vi "Begin.vi"() -> (0 "error out":errorcluster)   [LabVIEW 2013]
doc: "Called before other user functions, this VI is expected to open initial I/O refnums, load in file data, and do all program initialization. Notice that the <B>error out</B> terminal is simply used for data flow. Wiring it to other structures or subVIs ensures that this VI runs first."
uses:
  <vilib>/Rock Robotics/WPI/DriverStation/WPI_DriverStationRobotMode2.ctl
  <vilib>/Rock Robotics/WPI/Joystick/WPI_JoystickDeviceEnum.ctl
  <vilib>/Rock Robotics/SystemInterfaces/DIO/FPGA_DIOPWMChannel.ctl
  <vilib>/Rock Robotics/SystemInterfaces/DIO/FPGA_DIOChannel.ctl
  <vilib>/Rock Robotics/WPI/Encoder/WPI_EncoderType.ctl
  <vilib>/Rock Robotics/WPI/Solenoid/WPI_SolenoidChannel.ctl
  <vilib>/Rock Robotics/SystemInterfaces/AI/FPGA_AIGyroChannel.ctl
  <vilib>/Rock Robotics/SystemInterfaces/DIO/FPGA_DIORelayChannel.ctl
  Robot Global Data.vi
  <vilib>/Rock Robotics/WPI/Counter/WPI_CounterDigitalInputToDigitalSource.vi
  <vilib>/Rock Robotics/WPI/MotorControl/WPI_MotorControlOpen Talon.vi
  <vilib>/Rock Robotics/WPI/Solenoid/WPI_SolenoidOpenSingle.vi
  <vilib>/Rock Robotics/WPI/Compressor/WPI_CompressorGetSetRefNum.vi
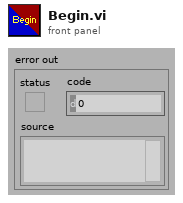
[diagram p1: front panel]
types:
  T1 = typedef "FPGA_DIORelayChannel.ctl" = enum8{"Relay 1", "Relay 2", "Relay 3", "Relay 4", "Relay 5", "Relay 6", "Relay 7", "Relay 8", "Invalid"}
  T2 = typedef "FPGA_DIOChannel.ctl" = enum8{"DIO 1", "DIO 2", "DIO 3", "DIO 4", "DIO 5", "DIO 6", "DIO 7", "DIO 8", "DIO 9", "DIO 10", "DIO 11", "DIO 12", "DIO 13", "DIO 14", "Invalid"}
  T3 = typedef "WPI_SolenoidChannel.ctl" = enum8{"Solenoid 1", "Solenoid 2", "Solenoid 3", "Solenoid 4", "Solenoid 5", "Solenoid 6", "Solenoid 7", "Solenoid 8", "Invalid"}
  T4 = typedef "FPGA_DIOPWMChannel.ctl" = enum8{"PWM 1", "PWM 2", "PWM 3", "PWM 4", "PWM 5", "PWM 6", "PWM 7", "PWM 8", "PWM 9", "PWM 10", "Invalid"}
  T5 = typedef "FPGA_AIGyroChannel.ctl" = enum8{"AI 1", "AI 2", "Invalid"}
  T6 = typedef "WPI_EncoderType.ctl" = enum16{"1x", "2x", "4x"}
  T7 = typedef "WPI_JoystickDeviceEnum.ctl" = enum16{"USB 1", "USB 2", "USB 3", "USB 4", "Kinect 1", "Kinect 2"}
  T8 = typedef "WPI_DriverStationRobotMode2.ctl" = enum16{"Autonomous Disabled", "Autonomous Enabled", "Teleop Disabled", "Teleop Enabled", "Timeout", "Finish", "Test Disabled", "Test Enabled"}
  T9 = typedef "WPI_JoystickDevRef.ctl" = cluster{"Device":T7}
  T10 = typedef "WPI_DigitalInputDevRef.ctl" = cluster{"DevStatus":errorcluster, "DIO Channel":T2, "Digital Module":T11}
  T11 = typedef "FPGA_TypedefDigitalModule.ctl" = enum16{"Digital Module 1", "Digital Module 2"}
  T12 = typedef "FPGA_CounterEncoderSourceConvertionLVSourceType.ctl" = cluster{"DevStatus":errorcluster, "AnalogTriggerMode?":bool, "DigitalMode":cluster{"Digital Module":T11, "DIO Channel":T13}, "AnalogTriggerMode":cluster{"AnalogTriggerIndex":T14, "OutputType":T15}}
  T13 = typedef "FPGA_DIODigitalSourceChannel.ctl" = enum8{"DIO 1", "DIO 2", "DIO 3", "DIO 4", "DIO 5", "DIO 6", "DIO 7", "DIO 8", "DIO 9", "DIO 10", "DIO 11", "DIO 12", "DIO 13", "DIO 14", "Disabled"}
  T14 = typedef "FPGA_AnalogTriggerIndex.ctl" = enum8{"Trig 0", "Trig 1", "Trig 2", "Trig 3", "Trig 4", "Trig 5", "Trig 6", "Trig 7", "Invalid"}
  T15 = typedef "FPGA_AnalogTriggerOutType.ctl" = enum16{"InWindow", "TriggerState", "Rising", "Falling"}
  T16 = typedef "WPI_EncoderDevRef.ctl" = cluster{"DevStatus":errorcluster, "EncoderIndex":T17, "CounterIndex":T18, "DistancePerCount":dbl, "Decoding Type":T6}
  T17 = typedef "FPGA_EncoderIdx.ctl" = enum8{"Enc 0", "Enc 1", "Enc 2", "Enc 3", "Invalid"}
  T18 = typedef "FPGA_CounterCtrSystemIndex.ctl" = enum8{"Ctr 0", "Ctr 1", "Ctr 2", "Ctr 3", "Ctr 4", "Ctr 5", "Ctr 6", "Ctr 7", "Invalid"}
  T19 = typedef "WPI_MotorControlDeviceRef.ctl" = cluster{"DeviceStatus":errorcluster, "Type":enum16{"PWM", "CAN"}, "PWM":cluster{"Digital Module":T11, "PWM Channel":T4, "DeadBand":T20}, "CAN":cluster{"Device Number":u8, "Control Mode":T21, "Semaphore":T22, "Max Vout":dbl}, "Invert":bool, "TransformRef":T23, "InvTransformRef":T23}
  T20 = typedef "WPI_PWMDeadband.ctl" = cluster{"Name":string, "maxPositivePwm":i32, "minPositivePwm":i32, "centerPwm":i32, "maxNegativePwm":i32, "minNegativePwm":i32, "angularRange":u16}
  T21 = typedef "WPI_CANJaguar_ControlMode.ctl" = enum8{"Percent VBus", "Current", "Speed", "Position", "Voltage"}
  T22 = typedef "Semaphore RefNum" = refnum<k1>
  T23 = typedef "WPI_PWMTransform_ConPane.ctl" = refnum<vi>
  T24 = typedef "WPI_GyroDevRef.ctl" = cluster{"DevStatus":errorcluster, "Analog Module":T25, "Analog Channel":T26, "Offset":dbl, "Gain (VoltsPerDegree/Second)":dbl}
  T25 = typedef "FPGA_TypedefAnalogModule.ctl" = enum16{"Analog Module 1", "Analog Module 2"}
  T26 = typedef "FPGA_AIChannel.ctl" = enum8{"AI 1", "AI 2", "AI 3", "AI 4", "AI 5", "AI 6", "AI 7", "AI 8", "Invalid"}
  T27 = typedef "WPI_SolenoidDevRef.ctl" = cluster{"DevStatus":errorcluster, "Solenoid Module":T28, "Forward Solenoid Channel":T3, "Reverse Solenoid Channel":T3}
  T28 = typedef "FPGA_TypedefSolenoidModule.ctl" = enum16{"Solenoid Module 1", "Solenoid Module 2"}
  T29 = typedef "WPI_CompressorDevRef.ctl" = cluster{"DevStatus":errorcluster, "DigitalInputDevRef":T10, "RelayDevRef":T30}
  T30 = typedef "WPI_RelayDevRef.ctl" = cluster{"DevStatus":errorcluster, "Relay Channel":T1, "Digital Module":T11, "Relay Direction":T31}
  T31 = typedef "WPI_RelayDirection.ctl" = enum16{"Both directions", "Forward only", "Reverse only"}
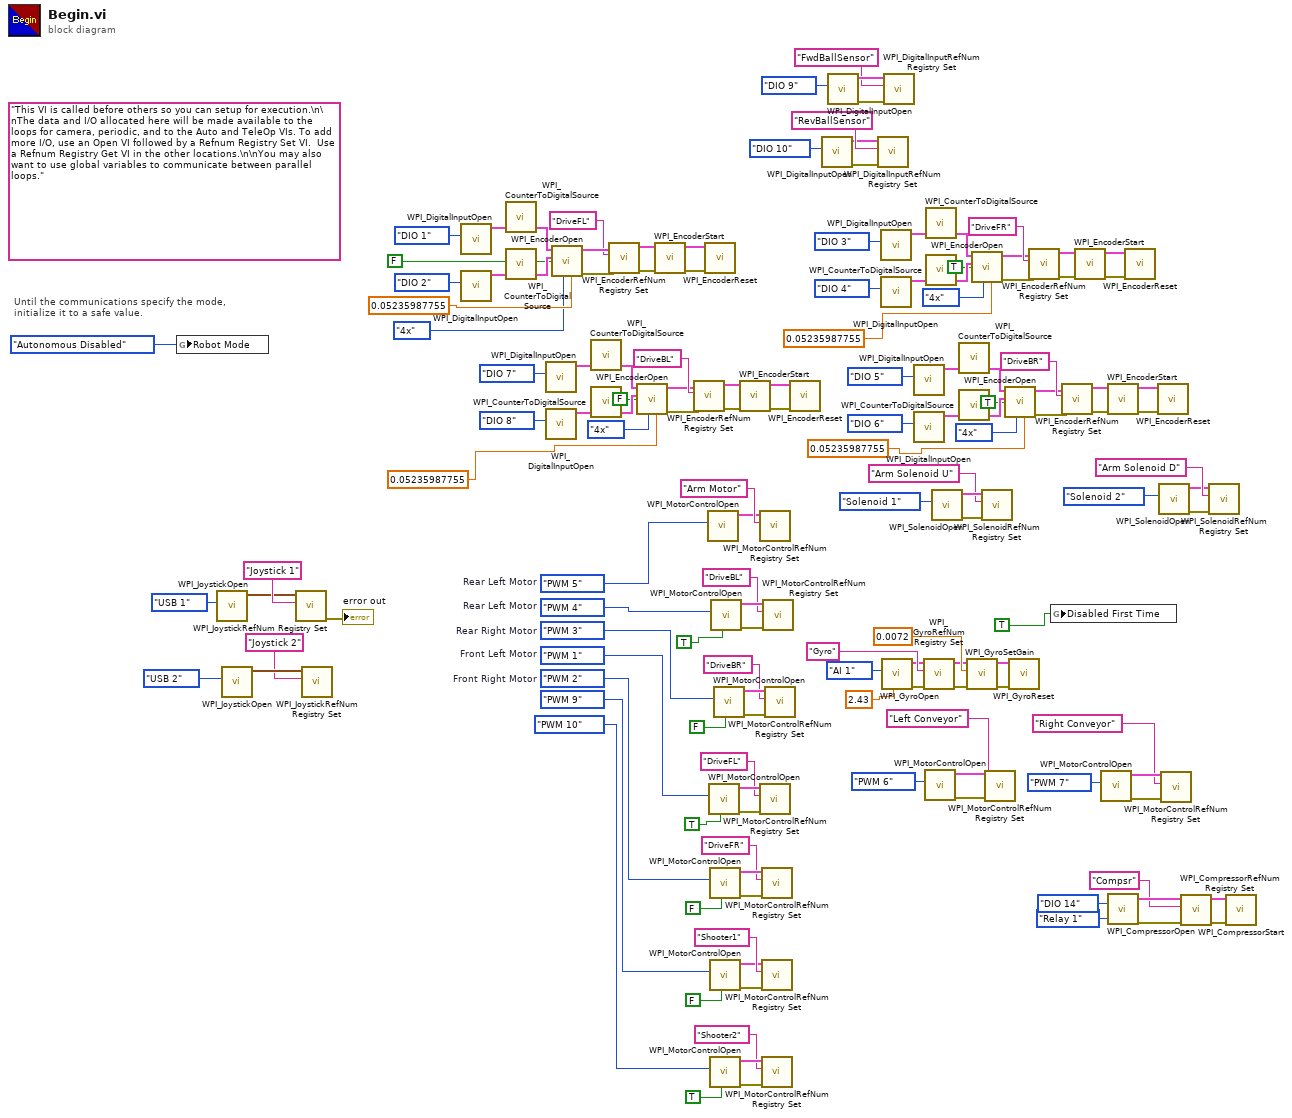
[diagram p0: block diagram]
diagram:
  w58 = FPGA_DIOPWMChannel."PWM 5"  # Rear Left Motor
  w67 = FPGA_DIOPWMChannel."PWM 2"  # Front Right Motor
  w68 = FPGA_DIOPWMChannel."PWM 1"  # Front Left Motor
  w69 = FPGA_DIOPWMChannel."PWM 3"  # Rear Right Motor
  w70 = FPGA_DIOPWMChannel."PWM 4"  # Rear Left Motor
  (unwired) "This VI is called before others so you can setup for execution.\n\nThe data and I/O allocated here will be made available to the loops for camera, periodic, and to the Auto and TeleOp VIs. To add more I/O, use an Open VI followed by a Refnum Registry Set VI.  Use a Refnum Registry Get VI in the other locations.\n\nYou may also want to use global variables to communicate between parallel loops."
  # "Until the communications specify the mode,\ninitialize it to a safe value."
  n1 = global write "Robot Global Data.vi" "Robot Mode"(WPI_DriverStationRobotMode2."Autonomous Disabled" ("Robot Mode")) -> ()
  n2 = call <vilib>:"WPI_JoystickOpen.vi"("JoystickDevice"=WPI_JoystickDeviceEnum."USB 1") -> ("JoystickDevRef"=w145:T9)  [unwired: 10 in]
  n3 = call <vilib>:"WPI_JoystickOpen.vi"("JoystickDevice"=WPI_JoystickDeviceEnum."USB 2") -> ("JoystickDevRef"=w141:T9)  [unwired: 10 in]
  n4 = call <vilib>:"WPI_JoystickRefNum Registry Set.vi"("refnum name"="Joystick 1", "JoystickDevRef"=w145) -> ("error out"=→"error out":errorcluster)  [unwired: 8 in, 1 out]
  n5 = call <vilib>:"WPI_JoystickRefNum Registry Set.vi"("refnum name"="Joystick 2", "JoystickDevRef"=w141) -> ()  [unwired: 8 in, 2 out]
  n6 = call <vilib>:"WPI_DigitalInputOpen.vi"("DIO Channel"=FPGA_DIOChannel."DIO 1") -> ("DigitalInputDevRef"=w113:T10)  [unwired: 9 in, 1 out]
  n7 = call <vilib>:"WPI_DigitalInputOpen.vi"("DIO Channel"=FPGA_DIOChannel."DIO 2") -> ("DigitalInputDevRef"=w116:T10)  [unwired: 9 in, 1 out]
  n8 = call-poly <vilib>:"WPI_CounterToDigitalSource.vi"("DigitalInputDevRef"=w113) -> ("Digital Source"=w114:T12)  [unwired: 6 in]
  n9 = call-poly <vilib>:"WPI_CounterToDigitalSource.vi"("DigitalInputDevRef"=w116) -> ("Digital Source"=w115:T12)  [unwired: 6 in]
  n10 = call <vilib>:"WPI_DigitalInputOpen.vi"("DIO Channel"=FPGA_DIOChannel."DIO 7") -> ("DigitalInputDevRef"=w137:T10)  [unwired: 9 in, 1 out]
  n11 = call <vilib>:"WPI_DigitalInputOpen.vi"("DIO Channel"=FPGA_DIOChannel."DIO 8") -> ("DigitalInputDevRef"=w134:T10)  [unwired: 9 in, 1 out]
  n12 = call <vilib>:"WPI_EncoderOpen.vi"("DistancePerCount"=0.05235987755, "Decoding Type"=WPI_EncoderType."4x", "Invert Direction (False)"=FALSE, "BSource"=w115, "ASource"=w114) -> ("error out"=w123:errorcluster, "EncoderDevRef"=w122:T16)  [unwired: 5 in]
  n13 = call-poly <vilib>:"WPI_CounterToDigitalSource.vi"("DigitalInputDevRef"=w137) -> ("Digital Source"=w136:T12)  [unwired: 6 in]
  n14 = call-poly <vilib>:"WPI_CounterToDigitalSource.vi"("DigitalInputDevRef"=w134) -> ("Digital Source"=w135:T12)  [unwired: 6 in]
  n15 = call <vilib>:"WPI_EncoderRefNum Registry Set.vi"("error in (no error)"=w123, "refnum name"="DriveFL", "EncoderDevRef"=w122) -> ("error out"=w125:errorcluster, "EncoderDevRef"=w124:T16)  [unwired: 7 in]
  n16 = call <vilib>:"WPI_EncoderOpen.vi"("DistancePerCount"=0.05235987755, "Decoding Type"=WPI_EncoderType."4x", "Invert Direction (False)"=FALSE, "BSource"=w135, "ASource"=w136) -> ("error out"=w128:errorcluster, "EncoderDevRef"=w129:T16)  [unwired: 5 in]
  n17 = call <vilib>:"WPI_EncoderStart.vi"("error in (no error)"=w125, "EncoderDevRef"=w124) -> ("error out"=w121:errorcluster, "EncoderDevRef"=w120:T16)  [unwired: 8 in]
  n18 = call <vilib>:"WPI_EncoderRefNum Registry Set.vi"("error in (no error)"=w128, "refnum name"="DriveBL", "EncoderDevRef"=w129) -> ("error out"=w126:errorcluster, "EncoderDevRef"=w127:T16)  [unwired: 7 in]
  n19 = call <vilib>:"WPI_EncoderReset.vi"("error in (no error)"=w121, "EncoderDevRef"=w120) -> ()  [unwired: 8 in, 2 out]
  n20 = call-poly <vilib>:"WPI_MotorControlOpen.vi"("PWM Channel"=w58) -> ("MotorControlDeviceRef"=w56:T19)  [unwired: 9 in, 1 out]
  n21 = call-poly <vilib>:"WPI_MotorControlOpen.vi"("Invert"=TRUE, "PWM Channel"=w68) -> ("error out"=w77:errorcluster, "MotorControlDeviceRef"=w78:T19)  [unwired: 8 in]
  n22 = call-poly <vilib>:"WPI_MotorControlOpen.vi"("Invert"=FALSE, "PWM Channel"=w67) -> ("error out"=w75:errorcluster, "MotorControlDeviceRef"=w76:T19)  [unwired: 8 in]
  n23 = call-poly <vilib>:"WPI_MotorControlOpen.vi"("Invert"=FALSE, "PWM Channel"=FPGA_DIOPWMChannel."PWM 9") -> ("error out"=w31:errorcluster, "MotorControlDeviceRef"=w30:T19)  [unwired: 8 in]
  n24 = call-poly <vilib>:"WPI_MotorControlOpen.vi"("Invert"=TRUE, "PWM Channel"=FPGA_DIOPWMChannel."PWM 10") -> ("error out"=w28:errorcluster, "MotorControlDeviceRef"=w29:T19)  [unwired: 8 in]
  n25 = call-poly <vilib>:"WPI_MotorControlOpen.vi"("Invert"=TRUE, "PWM Channel"=w70) -> ("error out"=w81:errorcluster, "MotorControlDeviceRef"=w82:T19)  [unwired: 8 in]
  n26 = call-poly <vilib>:"WPI_MotorControlOpen.vi"("Invert"=FALSE, "PWM Channel"=w69) -> ("error out"=w79:errorcluster, "MotorControlDeviceRef"=w80:T19)  [unwired: 8 in]
  n27 = call <vilib>:"WPI_EncoderStart.vi"("error in (no error)"=w126, "EncoderDevRef"=w127) -> ("error out"=w130:errorcluster, "EncoderDevRef"=w131:T16)  [unwired: 8 in]
  n28 = call <vilib>:"WPI_MotorControlRefNum Registry Set.vi"("refnum name"="Arm Motor", "MotorControlDevRef"=w56) -> ()  [unwired: 8 in, 2 out]
  n29 = call <vilib>:"WPI_MotorControlRefNum Registry Set.vi"("error in (no error)"=w77, "refnum name"="DriveFL", "MotorControlDevRef"=w78) -> ()  [unwired: 7 in, 2 out]
  n30 = call <vilib>:"WPI_MotorControlRefNum Registry Set.vi"("error in (no error)"=w75, "refnum name"="DriveFR", "MotorControlDevRef"=w76) -> ()  [unwired: 7 in, 2 out]
  n31 = call <vilib>:"WPI_MotorControlRefNum Registry Set.vi"("error in (no error)"=w31, "refnum name"="Shooter1", "MotorControlDevRef"=w30) -> ()  [unwired: 7 in, 2 out]
  n32 = call <vilib>:"WPI_MotorControlRefNum Registry Set.vi"("error in (no error)"=w28, "refnum name"="Shooter2", "MotorControlDevRef"=w29) -> ()  [unwired: 7 in, 2 out]
  n33 = call <vilib>:"WPI_MotorControlRefNum Registry Set.vi"("error in (no error)"=w81, "refnum name"="DriveBL", "MotorControlDevRef"=w82) -> ()  [unwired: 7 in, 2 out]
  n34 = call <vilib>:"WPI_MotorControlRefNum Registry Set.vi"("error in (no error)"=w79, "refnum name"="DriveBR", "MotorControlDevRef"=w80) -> ()  [unwired: 7 in, 2 out]
  n35 = call <vilib>:"WPI_EncoderReset.vi"("error in (no error)"=w130, "EncoderDevRef"=w131) -> ()  [unwired: 8 in, 2 out]
  n36 = call <vilib>:"WPI_DigitalInputOpen.vi"("DIO Channel"=FPGA_DIOChannel."DIO 10") -> ("error out"=w45:errorcluster, "DigitalInputDevRef"=w46:T10)  [unwired: 9 in]
  n37 = call <vilib>:"WPI_DigitalInputOpen.vi"("DIO Channel"=FPGA_DIOChannel."DIO 9") -> ("error out"=w50:errorcluster, "DigitalInputDevRef"=w49:T10)  [unwired: 9 in]
  n38 = call <vilib>:"WPI_DigitalInputRefNum Registry Set.vi"("error in (no error)"=w45, "refnum name"="RevBallSensor", "DigitalInputDevRef"=w46) -> ()  [unwired: 7 in, 2 out]
  n39 = call <vilib>:"WPI_DigitalInputOpen.vi"("DIO Channel"=FPGA_DIOChannel."DIO 3") -> ("DigitalInputDevRef"=w108:T10)  [unwired: 9 in, 1 out]
  n40 = call <vilib>:"WPI_DigitalInputOpen.vi"("DIO Channel"=FPGA_DIOChannel."DIO 4") -> ("DigitalInputDevRef"=w105:T10)  [unwired: 9 in, 1 out]
  n41 = call <vilib>:"WPI_GyroOpen.vi"("Calibrated Center Voltage"=2.43, "Analog Channel"=FPGA_AIGyroChannel."AI 1") -> ("error out"=w37:errorcluster, "GyroDevRef"=w36:T24)  [unwired: 7 in, 1 out]
  n42 = call <vilib>:"WPI_DigitalInputRefNum Registry Set.vi"("error in (no error)"=w50, "refnum name"="FwdBallSensor", "DigitalInputDevRef"=w49) -> ()  [unwired: 7 in, 2 out]
  n43 = call <vilib>:"WPI_DigitalInputOpen.vi"("DIO Channel"=FPGA_DIOChannel."DIO 5") -> ("DigitalInputDevRef"=w94:T10)  [unwired: 9 in, 1 out]
  n44 = call <vilib>:"WPI_DigitalInputOpen.vi"("DIO Channel"=FPGA_DIOChannel."DIO 6") -> ("DigitalInputDevRef"=w91:T10)  [unwired: 9 in, 1 out]
  n45 = call <vilib>:"WPI_GyroRefNum Registry Set.vi"("error in (no error)"=w37, "refnum name"="Gyro", "GyroDevRef"=w36) -> ("error out"=w38:errorcluster, "GyroDevRef"=w35:T24)  [unwired: 7 in]
  n46 = call-poly <vilib>:"WPI_MotorControlOpen.vi"("PWM Channel"=FPGA_DIOPWMChannel."PWM 6") -> ("error out"=w24:errorcluster, "MotorControlDeviceRef"=w23:T19)  [unwired: 9 in]
  n47 = call-poly <vilib>:"WPI_CounterToDigitalSource.vi"("DigitalInputDevRef"=w108) -> ("Digital Source"=w107:T12)  [unwired: 6 in]
  n48 = call-poly <vilib>:"WPI_CounterToDigitalSource.vi"("DigitalInputDevRef"=w105) -> ("Digital Source"=w106:T12)  [unwired: 6 in]
  n49 = call-poly <vilib>:"WPI_SolenoidOpen.vi"("Solenoid Channel"=WPI_SolenoidChannel."Solenoid 1") -> ("error out"=w54:errorcluster, "SolenoidDevRef"=w53:T27)  [unwired: 9 in]
  n50 = call-poly <vilib>:"WPI_CounterToDigitalSource.vi"("DigitalInputDevRef"=w94) -> ("Digital Source"=w93:T12)  [unwired: 6 in]
  n51 = call-poly <vilib>:"WPI_CounterToDigitalSource.vi"("DigitalInputDevRef"=w91) -> ("Digital Source"=w92:T12)  [unwired: 6 in]
  n52 = call <vilib>:"WPI_GyroSetGain.vi"("error in (no error)"=w38, "Gain (VoltsPerDegree/Second)"=0.0072, "GyroDevRef"=w35) -> ("error out"=w39:errorcluster, "GyroDevRef"=w34:T24)  [unwired: 7 in]
  n53 = call <vilib>:"WPI_EncoderOpen.vi"("DistancePerCount"=0.05235987755, "Decoding Type"=WPI_EncoderType."4x", "Invert Direction (False)"=TRUE, "BSource"=w106, "ASource"=w107) -> ("error out"=w99:errorcluster, "EncoderDevRef"=w100:T16)  [unwired: 5 in]
  n54 = call <vilib>:"WPI_SolenoidRefNum Registry Set.vi"("error in (no error)"=w54, "refnum name"="Arm Solenoid U", "SolenoidDevRef"=w53) -> ()  [unwired: 7 in, 2 out]
  n55 = call <vilib>:"WPI_MotorControlRefNum Registry Set.vi"("error in (no error)"=w24, "refnum name"="Left Conveyor", "MotorControlDevRef"=w23) -> ()  [unwired: 7 in, 2 out]
  n56 = call <vilib>:"WPI_EncoderOpen.vi"("DistancePerCount"=0.05235987755, "Decoding Type"=WPI_EncoderType."4x", "Invert Direction (False)"=TRUE, "BSource"=w92, "ASource"=w93) -> ("error out"=w85:errorcluster, "EncoderDevRef"=w86:T16)  [unwired: 5 in]
  n57 = call <vilib>:"WPI_GyroReset.vi"("error in (no error)"=w39, "GyroDevRef"=w34) -> ()  [unwired: 8 in, 2 out]
  n58 = call <vilib>:"WPI_EncoderRefNum Registry Set.vi"("error in (no error)"=w99, "refnum name"="DriveFR", "EncoderDevRef"=w100) -> ("error out"=w97:errorcluster, "EncoderDevRef"=w98:T16)  [unwired: 7 in]
  n59 = global write "Robot Global Data.vi" "Disabled First Time"(TRUE ("Disabled First Time")) -> ()
  n60 = call <vilib>:"WPI_EncoderRefNum Registry Set.vi"("error in (no error)"=w85, "refnum name"="DriveBR", "EncoderDevRef"=w86) -> ("error out"=w83:errorcluster, "EncoderDevRef"=w84:T16)  [unwired: 7 in]
  n61 = call <vilib>:"WPI_EncoderStart.vi"("error in (no error)"=w97, "EncoderDevRef"=w98) -> ("error out"=w101:errorcluster, "EncoderDevRef"=w102:T16)  [unwired: 8 in]
  n62 = call-poly <vilib>:"WPI_MotorControlOpen.vi"("PWM Channel"=FPGA_DIOPWMChannel."PWM 7") -> ("error out"=w21:errorcluster, "MotorControlDeviceRef"=w22:T19)  [unwired: 9 in]
  n63 = call <vilib>:"WPI_EncoderStart.vi"("error in (no error)"=w83, "EncoderDevRef"=w84) -> ("error out"=w87:errorcluster, "EncoderDevRef"=w88:T16)  [unwired: 8 in]
  n64 = call <vilib>:"WPI_CompressorOpen.vi"("Pressure Switch DIO Channel"=FPGA_DIOChannel."DIO 14", "Relay Channel"=FPGA_DIORelayChannel."Relay 1") -> ("CompressorDevRef"=w12:T29, "error out"=w6:errorcluster)  [unwired: 12 in]
  n65 = call <vilib>:"WPI_EncoderReset.vi"("error in (no error)"=w101, "EncoderDevRef"=w102) -> ()  [unwired: 8 in, 2 out]
  n66 = call <vilib>:"WPI_EncoderReset.vi"("error in (no error)"=w87, "EncoderDevRef"=w88) -> ()  [unwired: 8 in, 2 out]
  n67 = call-poly <vilib>:"WPI_SolenoidOpen.vi"("Solenoid Channel"=WPI_SolenoidChannel."Solenoid 2") -> ("error out"=w14:errorcluster, "SolenoidDevRef"=w15:T27)  [unwired: 9 in]
  n68 = call <vilib>:"WPI_MotorControlRefNum Registry Set.vi"("error in (no error)"=w21, "refnum name"="Right Conveyor", "MotorControlDevRef"=w22) -> ()  [unwired: 7 in, 2 out]
  n69 = call <vilib>:"WPI_CompressorRefNum Registry Set.vi"("error in (no error)"=w6, "refnum name"="Compsr", "CompressorDevRef"=w12) -> ("error out"=w8:errorcluster, "CompressorDevRef"=w7:T29)  [unwired: 7 in]
  n70 = call <vilib>:"WPI_SolenoidRefNum Registry Set.vi"("error in (no error)"=w14, "refnum name"="Arm Solenoid D", "SolenoidDevRef"=w15) -> ()  [unwired: 7 in, 2 out]
  n71 = call <vilib>:"WPI_CompressorStart.vi"("error in (no error)"=w8, "CompressorDevRef"=w7) -> ()  [unwired: 8 in, 2 out]
